vi "APS arc2 ce all.vi"(0 "Axis_ID_Array":i32, 1 "Option":i32, 2 "CenterArray":dbl, 3 "EndArray":dbl, 4 "Dir":i16, 5 "TransPara":dbl, 6 "Vs":dbl, 7 "error in (no error)":errorcluster caption="错误输入（无错误）", 8 "Vm":dbl, 9 "Ve":dbl, 10 "Acc":dbl, 11 "Dec":dbl, 12 "SFac":dbl, 13 "Wait":cluster{"h_event":u32, "i32_ret":i32}) -> (15 "Wait out":cluster{"h_event":u32, "i32_ret":i32}, 20 "Axis_ID_Array out":i32, 21 "function return":i32, 22 "CenterArray out":dbl, 23 "EndArray out":dbl, 25 "TransPara out":dbl, 27 "error out":errorcluster caption="错误输出")   [LabVIEW 2011, in "APS168.lvlib"]
doc: "I32 FNTYPE APS_arc2_ce_all( I32 *Axis_ID_Array, I32 Option, F64 *CenterArray, F64 *EndArray, I16 Dir, F64 *TransPara, F64 Vs, F64 Vm, F64 Ve, F64 Acc,F64 Dec, F64 SFac, ASYNCALL *Wait );"
uses:
  APS168.lvlib
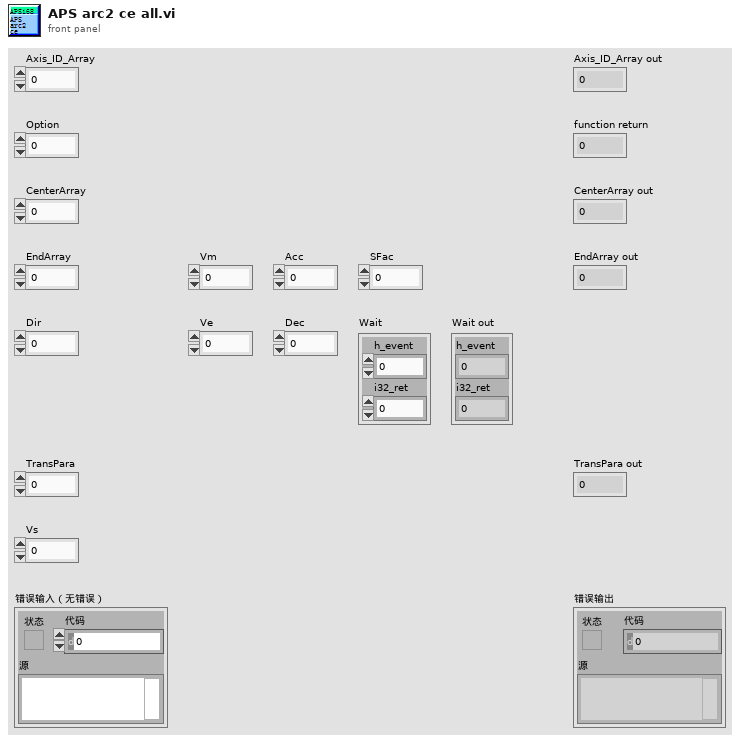
[diagram p1: front panel]
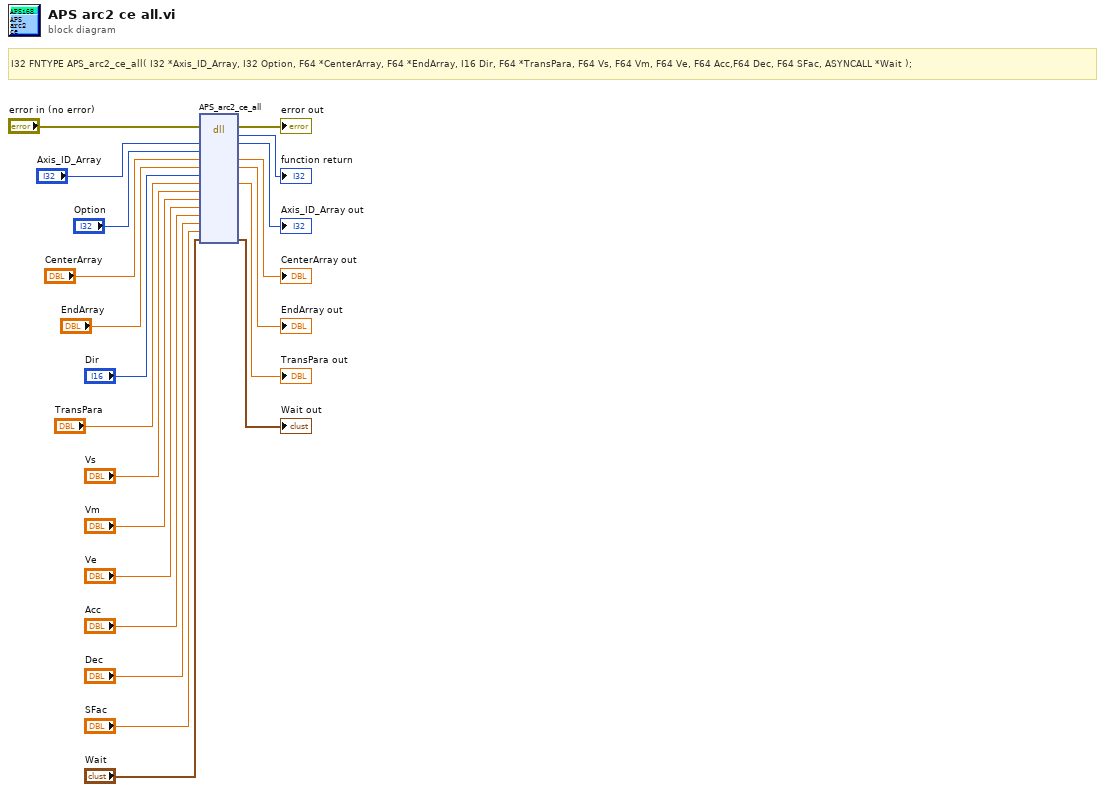
[diagram p0: block diagram]
diagram:
  # "I32 FNTYPE APS_arc2_ce_all( I32 *Axis_ID_Array, I32 Option, F64 *CenterArray, F64 *EndArray, I16 Dir, F64 *TransPara, F64 Vs, F64 Vm, F64 Ve, F64 Acc,F64 Dec, F64 SFac, ASYNCALL *Wait );"
  n1 = dll-call lib="PTH1Labs E软件ADLINK 204CAPS_1_7_1_LIB line 连续运动204APS168.*" fn="APS_arc2_ce_all"(error in="error in (no error)", "Axis_ID_Array"="Axis_ID_Array", "Option"="Option", "CenterArray"="CenterArray", "EndArray"="EndArray", "Dir"="Dir", "TransPara"="TransPara", "Vs"="Vs", "Vm"="Vm", "Ve"="Ve", "Acc"="Acc", "Dec"="Dec", "SFac"="SFac", "Wait"="Wait") -> (error out=→"error out":errorcluster, →"function return":i32, "Axis_ID_Array"=→"Axis_ID_Array out":i32, "CenterArray"=→"CenterArray out":dbl, "EndArray"=→"EndArray out":dbl, "TransPara"=→"TransPara out":dbl, "Wait"=→"Wait out":cluster{"h_event":u32, "i32_ret":i32})  [unwired: 10 in, 1 out]
